vi "Serial_WrRd.vi"(5 "ReadInterval(mSec)":u32=75, 7 "Timeout(Sec)":dbl=5.0, 8 "error in (no error)":errorcluster, 9 "PassString":string="PASS", 10 "Command":string, 11 "ComPort":refnum<visa-resource-name>="COM10") -> (0 "error out":errorcluster, 2 "PASS":bool, 3 "received":string)   [LabVIEW 2018]
uses:
  <vilib>/Instr/_visa.llb/VISA Configure Serial Port (Instr).vi
panel:
  out "concatenated string":string
  # "ADB Serial W/R"
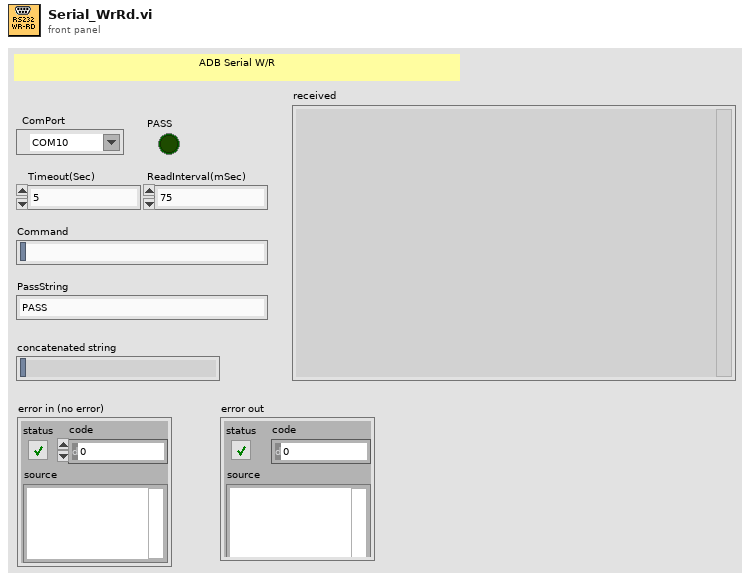
[diagram p1: front panel]
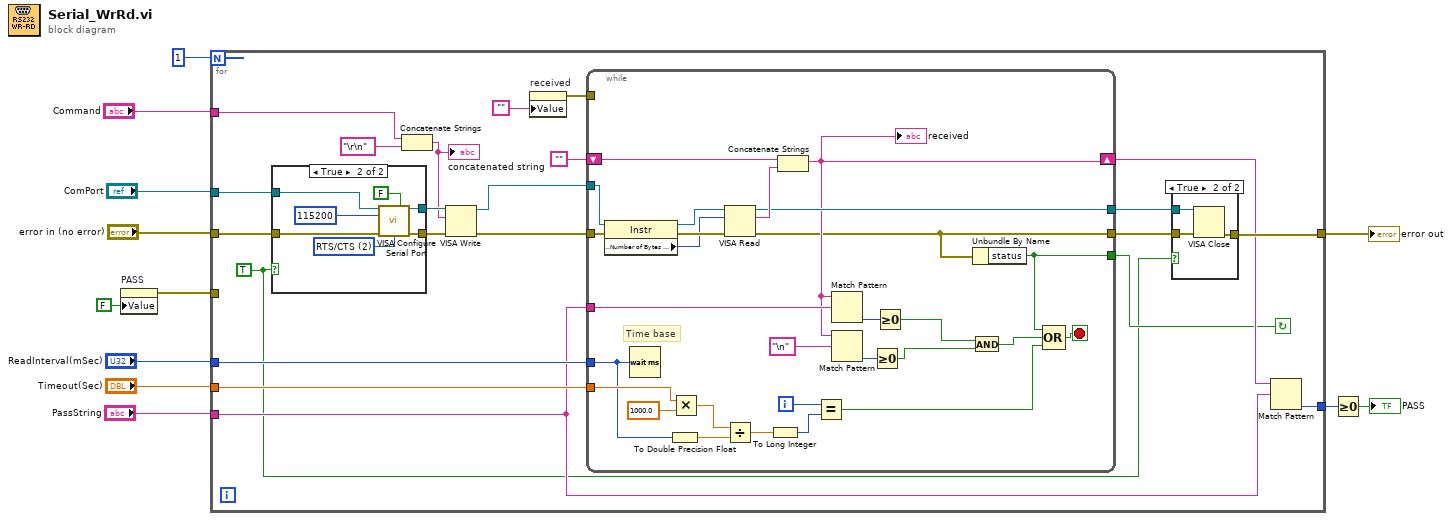
[diagram p0: block diagram]
diagram:
  n1 = property on="PASS" class="Bool (strict)"("Value"=FALSE ("PASS")) -> (error out=w2:errorcluster)  [unwired: 2 in, 1 out]
  n2 = for {
    N: 1 -> [_]
    tunnel: "ComPort" -> [w34]
    tunnel: "ReadInterval(mSec)" -> [w33]
    tunnel: [w32] -> w9
    tunnel: "Timeout(Sec)" -> [w28]
    tunnel: "PassString" -> [w22]
    tunnel: "Command" -> [w18]
    tunnel: "error in (no error)" -> [w31]
    tunnel: [w27] -> w3
    tunnel: w2 -> [_]
    stop <- w14 continue-if-true
    w13 = TRUE
    n3 = case shown="True" w13 {
      tunnel: w34 -> [w40 w47]
      tunnel: w31 -> [w39 w46]
      tunnel: [w40 w44] -> w30
      tunnel: [w39 w43] -> w29
      frame False {
      }
      frame True {
        w41 = u16 2 items=["None", "XON/XOFF", "RTS/CTS", "XON/XOFF & RTS/CTS", "DTR/DSR", "XON/XOFF & DTR/DSR"] ("flow control (0:none)")
        n4 = call-poly "VISA Configure Serial Port"("VISA resource name"=w47, "Enable Termination\nChar (T)"=FALSE ("Enable Termination\nChar (T)"), "baud rate (9600)"=u32 115200 ("Serial Settings:Baud Rate"), "error in (no error)"=w46, "flow control (0:none)"=w41) -> ("VISA resource name out"=w44:refnum<visa-resource-name>, "error out"=w43:errorcluster)  [unwired: 9 in]
      }
    }
    n5 = Concatenate Strings(w18, "\r\n" ("string")) -> (w19:string)
    "concatenated string" <- w19
    n6 = VISA Write(VISA resource name=w30, write buffer=w19, error in (no error)=w29) -> (VISA resource name out=w23:refnum<visa-resource-name>, error out=w15:errorcluster)  [unwired: 1 out]
    n7 = property on="received" class="Str"("Value"="") -> (error out=w16:errorcluster)  [unwired: 2 in, 1 out]
    n8 = while {
      tunnel: w15 -> [w75]
      tunnel: w23 -> [w74]
      tunnel: [w49] -> w25
      shift-right: [w53] -> w20
      shift-left: "" -> [w71]
      tunnel: [w69] -> w26
      tunnel: w33 -> [w62]
      tunnel: w28 -> [w65]
      tunnel: w22 -> [w56]
      tunnel: [w48] -> w14
      tunnel: w16 -> [_]
      i -> [w66]
      stop <- w68 stop-if-true
      # "Time base"
      n9 = property class="Instr"(reference=w74, error in=w75) -> (reference out=w72:refnum<visa-resource-name>, error out=w73:errorcluster, "Serial Settings:Number of Bytes at Serial Port"=w58:u32)
      n10 = Wait (ms)(milliseconds to wait=w62) -> ()  [unwired: 1 out]
      n11 = To Double Precision Float(number=w62) -> (double precision float=w59:dbl)
      n12 = Multiply(x=w65, y=1000.0) -> (x*y=w63:dbl)
      n13 = VISA Read(VISA resource name=w72, byte count=w58, error in (no error)=w73) -> (VISA resource name out=w69:refnum<visa-resource-name>, read buffer=w70:string, error out=w49:errorcluster)  [unwired: 1 out]
      n14 = Divide(x=w63, y=w59) -> (x/y=w61:dbl)
      n15 = To Long Integer(number=w61) -> (32bit integer=w60:i32)
      n16 = Concatenate Strings(w71, w70) -> (w53:string)
      "received" <- w53
      n17 = Equal?(x=w66, y=w60) -> (x = y?=w67:bool)
      n18 = Match Pattern(string=w53, regular expression=w56) -> (offset past match=w57:i32)  [unwired: 1 in, 3 out]
      n19 = Match Pattern(string=w53, regular expression="\n") -> (offset past match=w55:i32)  [unwired: 1 in, 3 out]
      n20 = Greater Or Equal To 0?(x=w55) -> (x >= 0?=w50:bool)
      n21 = Greater Or Equal To 0?(x=w57) -> (x >= 0?=w51:bool)
      n22 = And(x=w51, y=w50) -> (x .and. y?=w54:bool)
      n23 = Unbundle By Name(w49) -> ("status"=w48:bool)
      n24 = Compound Arithmetic op=OR(w48, w54, w67) -> (w68:bool)
    }
    n25 = case shown="True" w13 {
      tunnel: [w35 w38] -> w27
      tunnel: w26 -> [_ w37]
      tunnel: w25 -> [w35 w36]
      frame False {
      }
      frame True {
        n26 = VISA Close(VISA resource name=w37, error in (no error)=w36) -> (error out=w38:errorcluster)
      }
    }
    n27 = Match Pattern(string=w20, regular expression=w22) -> (offset past match=w32:i32)  [unwired: 1 in, 3 out]
  }
  "error out" <- w3
  n28 = Greater Or Equal To 0?(x=w9) -> (x >= 0?=→"PASS":bool)
